vi "EditItem.vi"(8 "Error":errorcluster, 9 "EditData":cluster{"Strings":string[], "Variant":variant}, 10 "Tag":string, 11 "Tree in":refnum<class "Tree.lvclass">) -> (0 "Error":errorcluster, 1 "ItemData":T1, 2 "Found?":bool, 3 "Tree out":refnum<class "Tree.lvclass">)   [LabVIEW 2021, in "Tree.lvlib" / "Tree.lvclass"]
uses:
  Tree.lvclass
  Private/TreeControllerTag.ctl
  Tree.lvclass/Tree.ctl
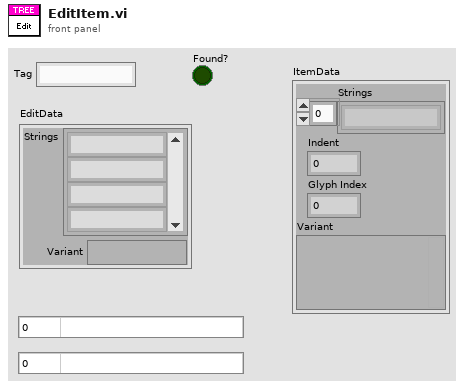
[diagram p1: front panel]
types:
  T1 = cluster{"Strings":string[], "Indent":i32, "Glyph Index":i32, "Variant":variant}
  T2 = cluster{"Found":bool, "ItemData":cluster{"Strings":string[], "Indent":i32, "Glyph Index":i32, "Variant":variant}}
  T3 = typedef "Tree.lvlib/Tree.lvclass/TreeControllerTag.ctl" = enum8{"Null", "1. Add item", "2. Delete item", "3. Get All Tree Data", "4. Drag Starting", "5. Drag Ended", "6. Add Tree Values", "7. Get Item Value", "8. Edit Item", "9. StepBack", "10. Filter"}
  T4 = cluster{"Tag":string, "Strings":string[], "Variant":variant}
  T5 = cluster{"NewElement":cluster{"Tag":string, "Strings":string[], "Variant":variant}, "queue out":refnum<queue>}
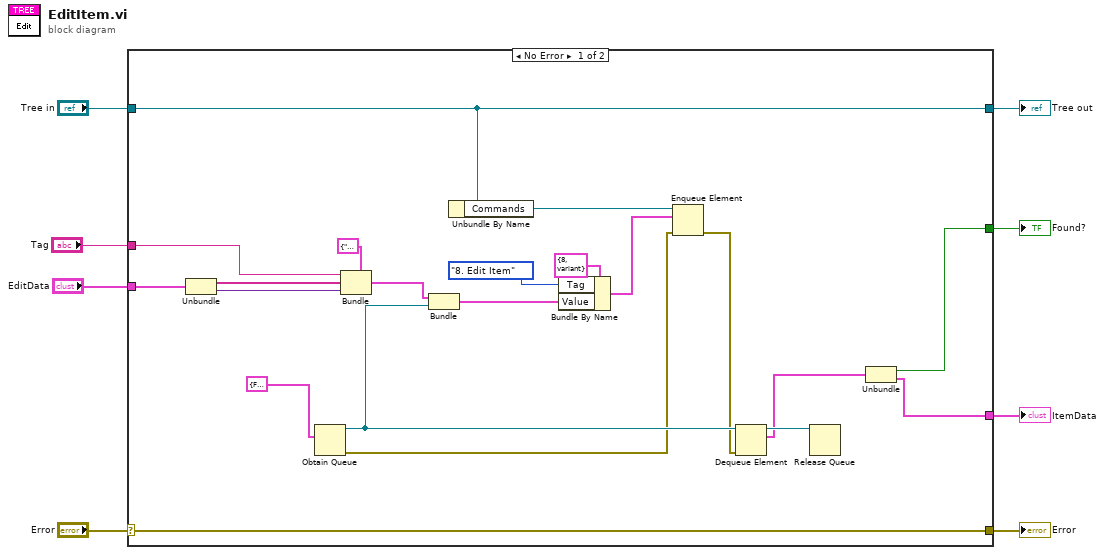
[diagram p0: block diagram]
diagram:
  n1 = case shown="No Error" "Error" {
    selector: "Error" -> [w29 w31]
    tunnel: [w29 w31] -> w7
    tunnel: [w28 w30] -> w5
    tunnel: "Tree in" -> [w28 w30]
    tunnel: "EditData" -> [w18 _]
    tunnel: [w12 _] -> w3
    tunnel: "Tag" -> [w19 _]
    tunnel: [w11 _] -> w1
    frame No Error {
      n2 = Unbundle(w18) -> ("Strings"=w17:string[], "Variant"=w16:variant)
      n3 = Obtain Queue(element data type=T2 {"Found"=FALSE, "ItemData"={"Strings"=[], "Indent"=0, "Glyph Index"=0, "Variant"=variant}} ("output cluster")) -> (queue out=w23:refnum<queue>, error out=w9:errorcluster)  [unwired: 4 in, 1 out]
      n4 = Bundle(cluster=T4 {"Tag"="", "Strings"=[], "Variant"=variant} ("NewElement"), "Tag"=w19, "Strings"=w17, "Variant"=w16) -> (w20:T4)
      n5 = Bundle("NewElement"=w20, "queue out"=w23) -> (w24:T5)  [unwired: 1 in]
      n6 = Unbundle By Name(w28) -> ("Commands"=w27:refnum<queue>)
      n7 = Bundle By Name(cluster=cluster{"Tag":u8, "Value":variant} {"Tag"=8, "Value"=variant} ("element"), "Tag"=TreeControllerTag."8. Edit Item", "Value"=w24) -> (w25:cluster{"Tag":u8, "Value":variant})
      n8 = Enqueue Element(queue=w27, element=w25, error in (no error)=w9) -> (error out=w10:errorcluster)  [unwired: 1 in, 2 out]
      n9 = Dequeue Element(queue=w23, error in (no error)=w10) -> (queue out=w22:refnum<queue>, element=w13:T2)  [unwired: 1 in, 2 out]
      n10 = Release Queue(queue=w22) -> ()  [unwired: 2 in, 3 out]
      n11 = Unbundle(w13) -> ("Found"=w12:bool, "ItemData"=w11:T1)
    }
    frame Error {
    }
  }
  "Error" <- w7
  "Tree out" <- w5
  "Found?" <- w3
  "ItemData" <- w1
